vi "ASDDark.vi"(0 "TCP Network Connection Refnum":refnum<k5>, 7 "Collect Dark":bool, 11 "error in (no error)":errorcluster) -> (4 "Header Code":i32, 6 "Error Code":i32, 8 "Dark Corrected Spectrum Data":dbl[](array[numeric]), 15 "error out":errorcluster)   [LabVIEW 2010]
uses:
  Instance           4 15Saved   ASDDark .vi
panel:
  # "This is a Sub-VI of ASDTCPDemo."
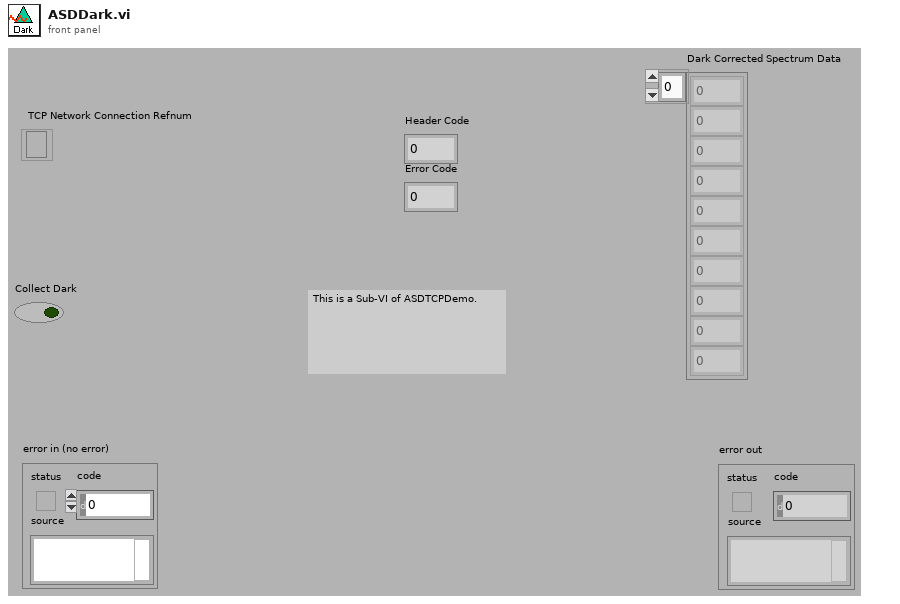
[diagram p1: front panel]
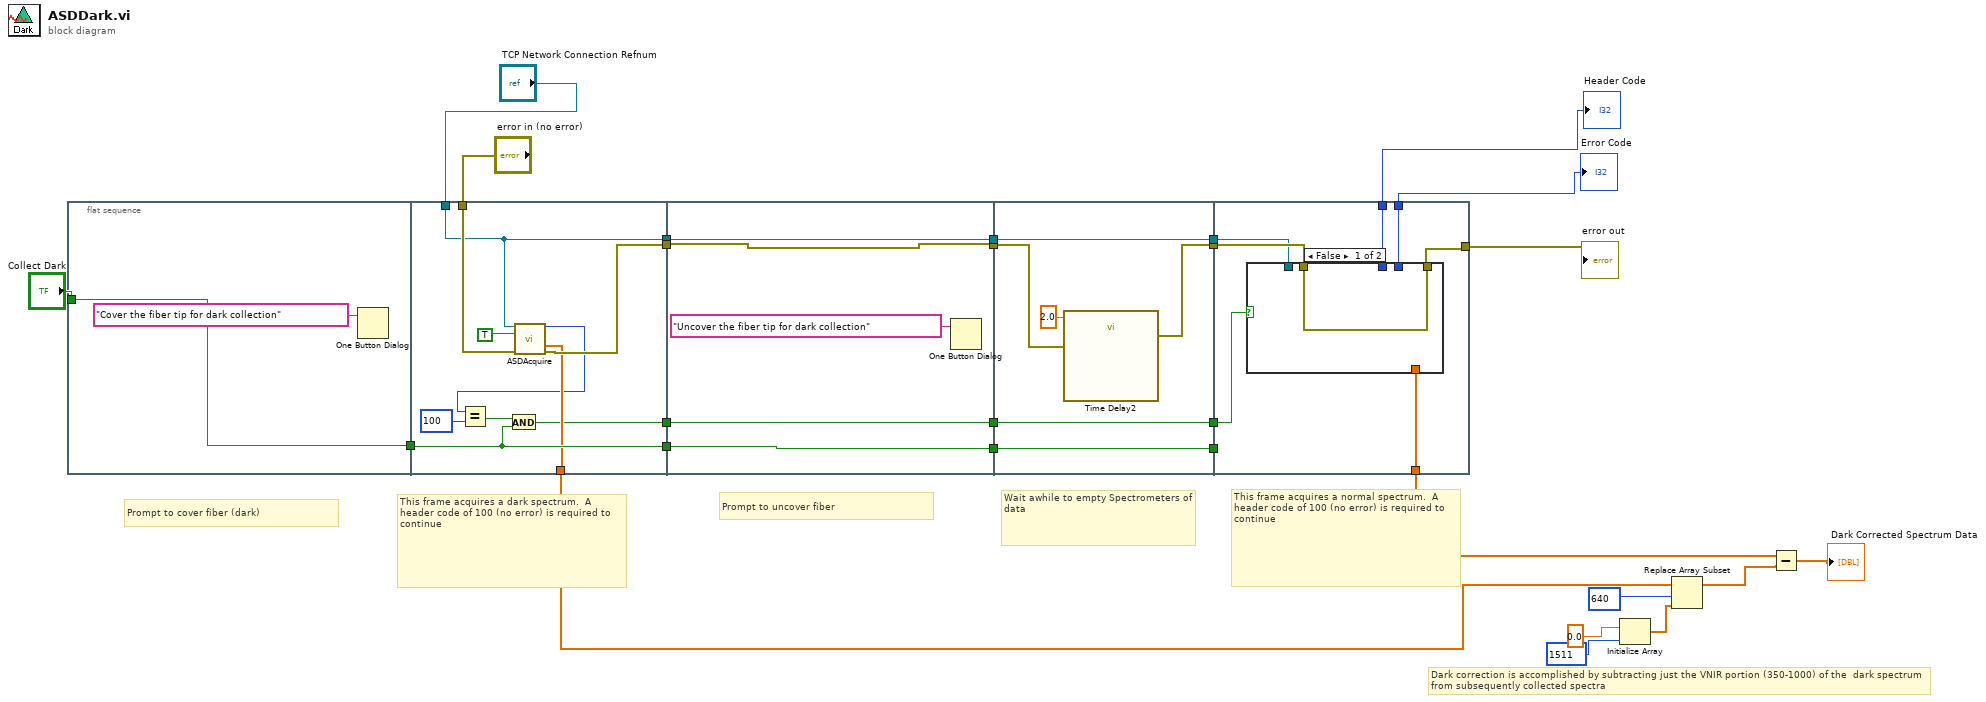
[diagram p0: block diagram]
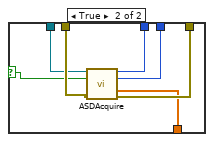
[diagram p2: hidden frame]
diagram:
  # "Prompt to uncover fiber"
  # "Wait awhile to empty Spectrometers of data"
  # "Dark correction is accomplished by subtracting just the VNIR portion (350-1000) of the  dark spectrum from subsequently collected spectra"
  # "This frame acquires a normal spectrum.  A header code of 100 (no error) is required to\ncontinue"
  # "This frame acquires a dark spectrum.  A header code of 100 (no error) is required to\ncontinue"
  # "Prompt to cover fiber (dark)"
  n1 = flat-sequence {
    tunnel: [w29] -> w7
    tunnel: "Collect Dark" -> [w29]
    tunnel: [w30] -> w26
    tunnel: [w34] -> w15
    tunnel: w7 -> [w37]
    tunnel: [w37] -> w25
    tunnel: "error in (no error)" -> [w36]
    tunnel: [w35] -> w5
    tunnel: [w32] -> w2
    tunnel: "TCP Network Connection Refnum" -> [w30]
    tunnel: [w41] -> w21
    tunnel: w26 -> [w43]
    tunnel: [w43] -> w20
    tunnel: w25 -> [w44]
    tunnel: [w44] -> w18
    tunnel: w5 -> [w41]
    tunnel: [w42] -> w3
    tunnel: w2 -> [w42]
    tunnel: w21 -> [w47]
    tunnel: w20 -> [w50]
    tunnel: [w50] -> w19
    tunnel: w18 -> [w49]
    tunnel: [w49] -> w17
    tunnel: [w46] -> w16
    tunnel: [w45] -> w4
    tunnel: w3 -> [w45]
    tunnel: [w57] -> w27
    tunnel: w16 -> [w56]
    tunnel: w19 -> [w55]
    tunnel: [w54] -> w14
    tunnel: [w52] -> w22
    tunnel: [w53] -> w23
    tunnel: w17 -> [_]
    tunnel: w4 -> [w51]
    frame #0 {
      n2 = One Button Dialog(message="Cover the fiber tip for dark collection") -> ()  [unwired: 1 in, 1 out]
    }
    frame #1 {
      n3 = call "ASDAcquire.vi"("TCP Network Connection Refnum"=w30, "Acquire"=TRUE, "error in (no error)"=w36) -> ("Header Code"=w31:i32, "Spectrum Data"=w34:sgl[], "error out"=w35:errorcluster)  [unwired: 9 in, 1 out]
      n4 = Equal?(x=w31, y=100) -> (x = y?=w38:bool)
      n5 = And(x=w38, y=w37) -> (x .and. y?=w32:bool)
    }
    frame #2 {
      n6 = One Button Dialog(message="Uncover the fiber tip for dark collection") -> ()  [unwired: 1 in, 1 out]
    }
    frame #3 {
      n7 = call "Time Delay2"("error in (no error)"=w47, "Delay Time (s)"=2.0) -> ("error out"=w46:errorcluster)  [unwired: 9 in]
    }
    frame #4 {
      n8 = case shown="False" w51 {
        selector: w51 -> [_ w59]
        tunnel: [w58 w65] -> w57
        tunnel: w56 -> [w58 w64]
        tunnel: w55 -> [_ w63]
        tunnel: [_ w62] -> w54
        tunnel: [_ w61] -> w52
        tunnel: [_ w60] -> w53
        frame False {
        }
        frame True {
          n9 = call "ASDAcquire.vi"("TCP Network Connection Refnum"=w63, "Acquire"=w59, "error in (no error)"=w64) -> ("Header Code"=w61:i32, "Error Code"=w60:i32, "Spectrum Data"=w62:sgl[], "error out"=w65:errorcluster)  [unwired: 9 in]
        }
      }
    }
  }
  n10 = Initialize Array(0.0 ("element"), 1511 ("dimension size")) -> (w8:dbl[])
  n11 = Replace Array Subset(array=w15, new element=w8, index=640) -> (w13:sgl[])
  n12 = Subtract(x=w14, y=w13) -> (x-y=→"Dark Corrected Spectrum Data":sgl[])
  "error out" <- w27
  "Header Code" <- w22
  "Error Code" <- w23
